vi "Arduino read multiple 10times resolution Feb2017.vi"(5 "# of points to average":i32, 8 "arduino addresses in":T2, 9 "average points?":bool, 10 "arduinos on?":bool) -> (1 "arduino addresses out":T2, 2 "freq out":T1, 3 "arduinos on":bool)   [LabVIEW 2014]
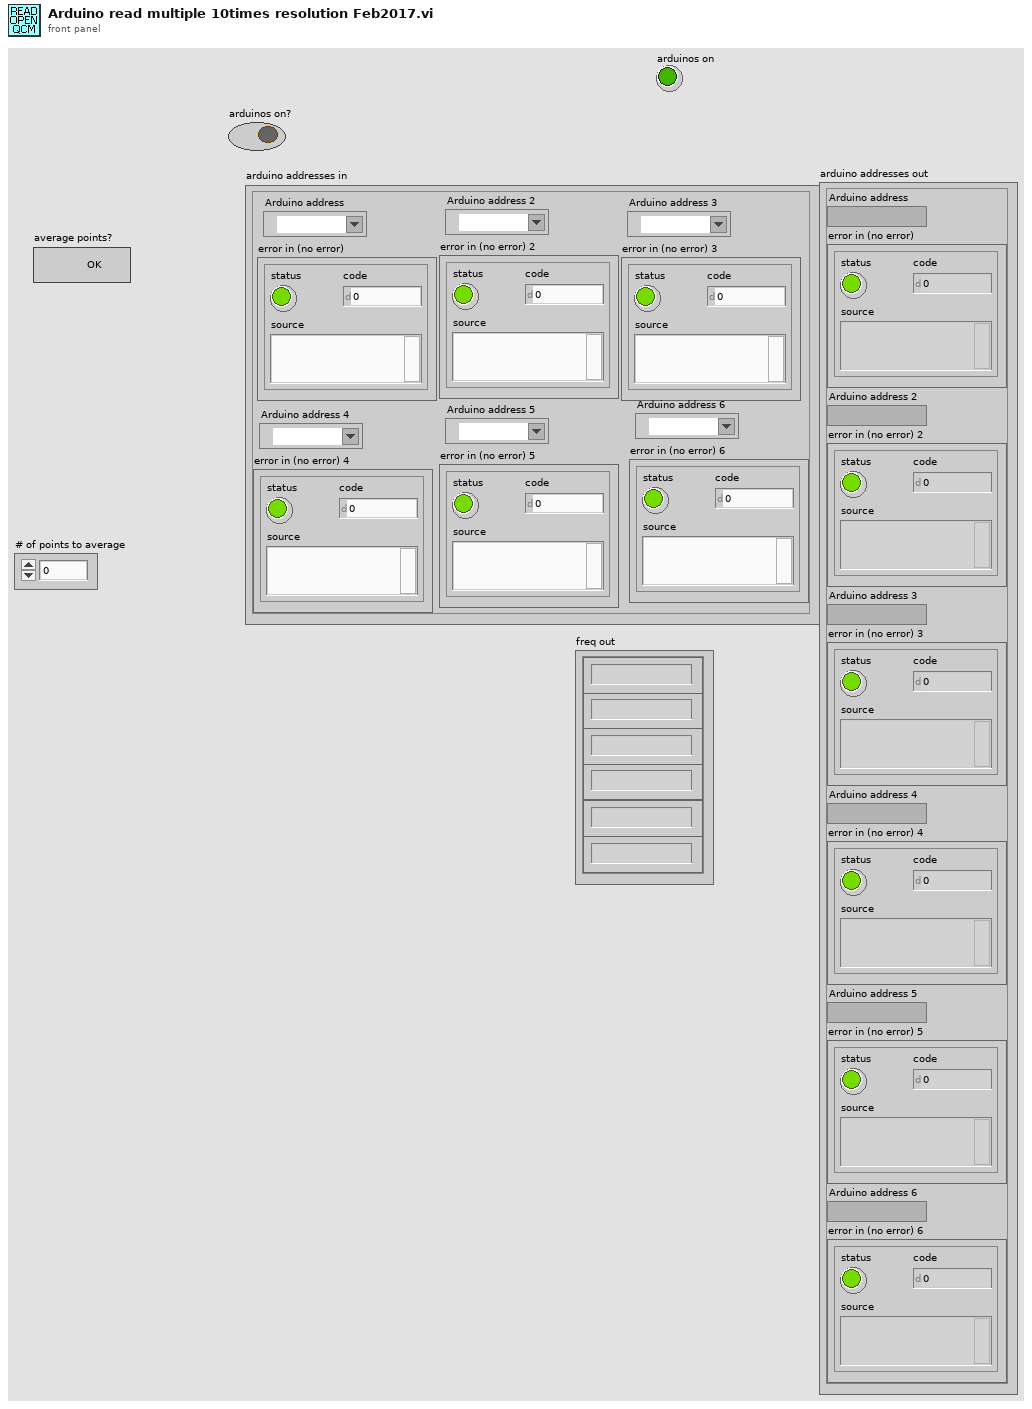
[diagram p1: front panel]
types:
  T1 = cluster{"String":string, "String":string, "String":string, "String":string, "String":string, "String":string}
  T2 = cluster{"Arduino address":refnum<visa-resource-name>, "error in (no error)":errorcluster, "Arduino address 2":refnum<visa-resource-name>, "error in (no error) 2":errorcluster, "Arduino address 3":refnum<visa-resource-name>, "error in (no error) 3":errorcluster, "Arduino address 4":refnum<visa-resource-name>, "error in (no error) 4":errorcluster, "Arduino address 5":refnum<visa-resource-name>, "error in (no error) 5":errorcluster, "Arduino address 6":refnum<visa-resource-name>, "error in (no error) 6":errorcluster}
  T3 = cluster{string, string, string, string, string, string}
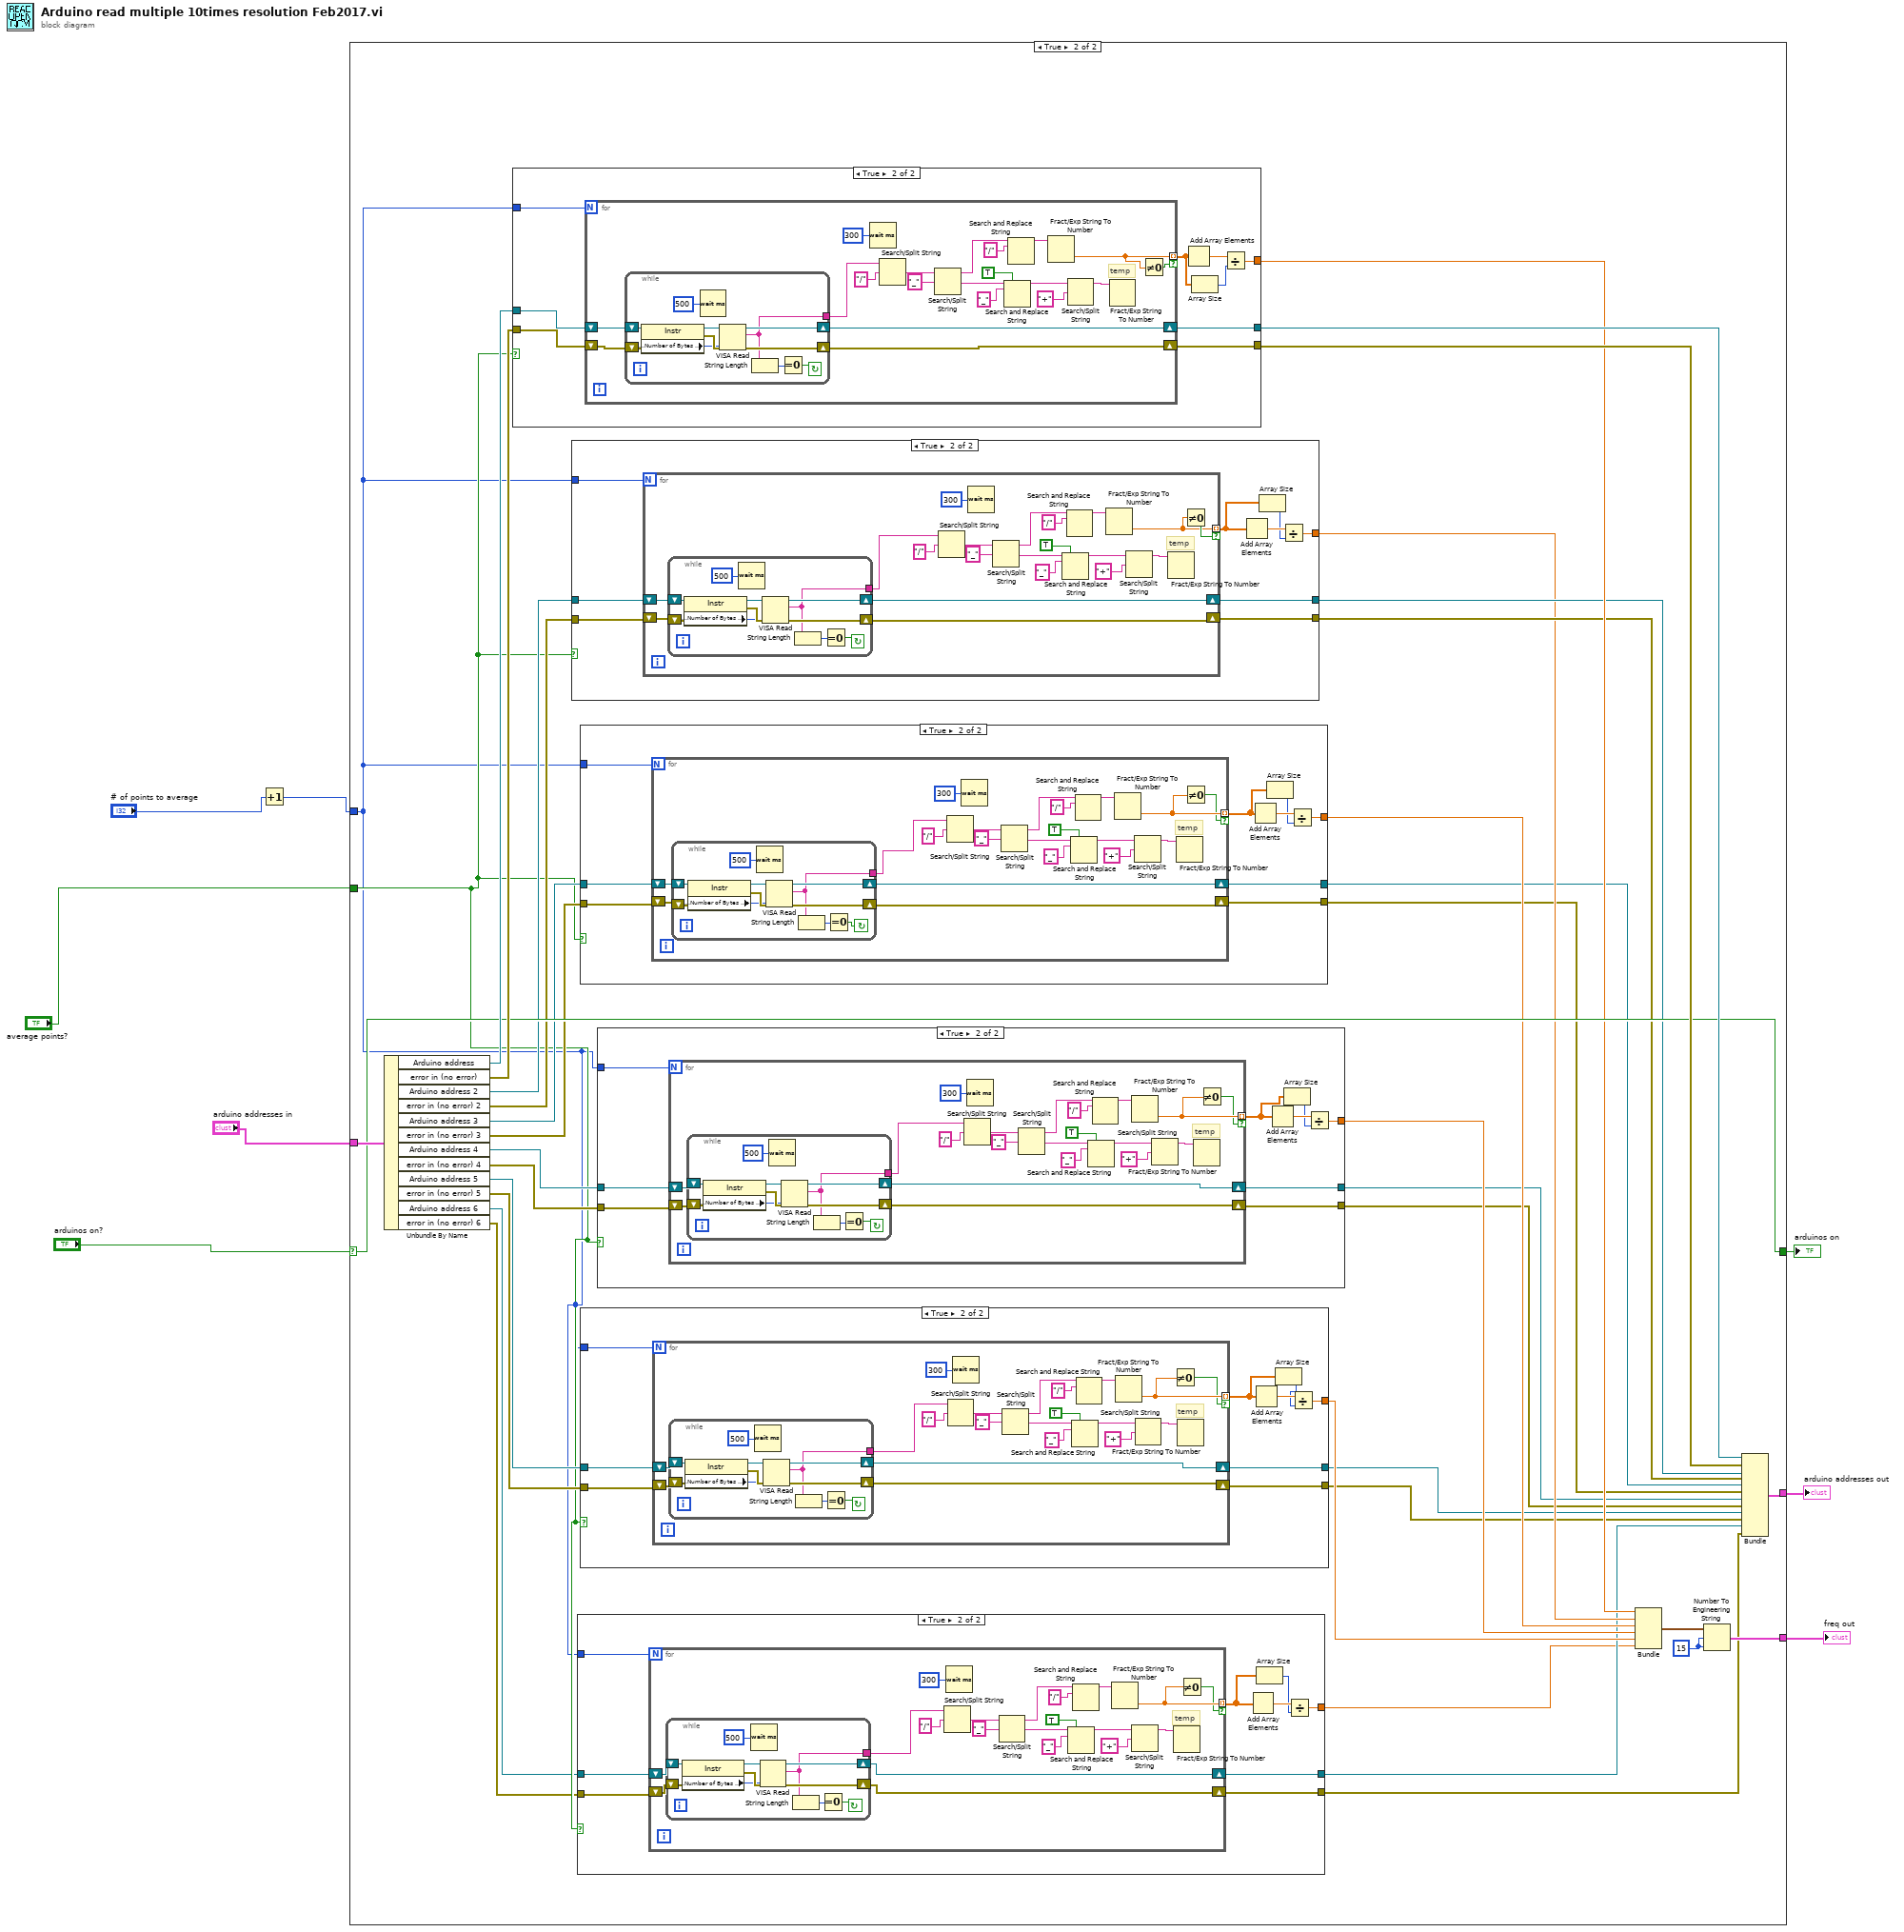
[diagram p0: block diagram]
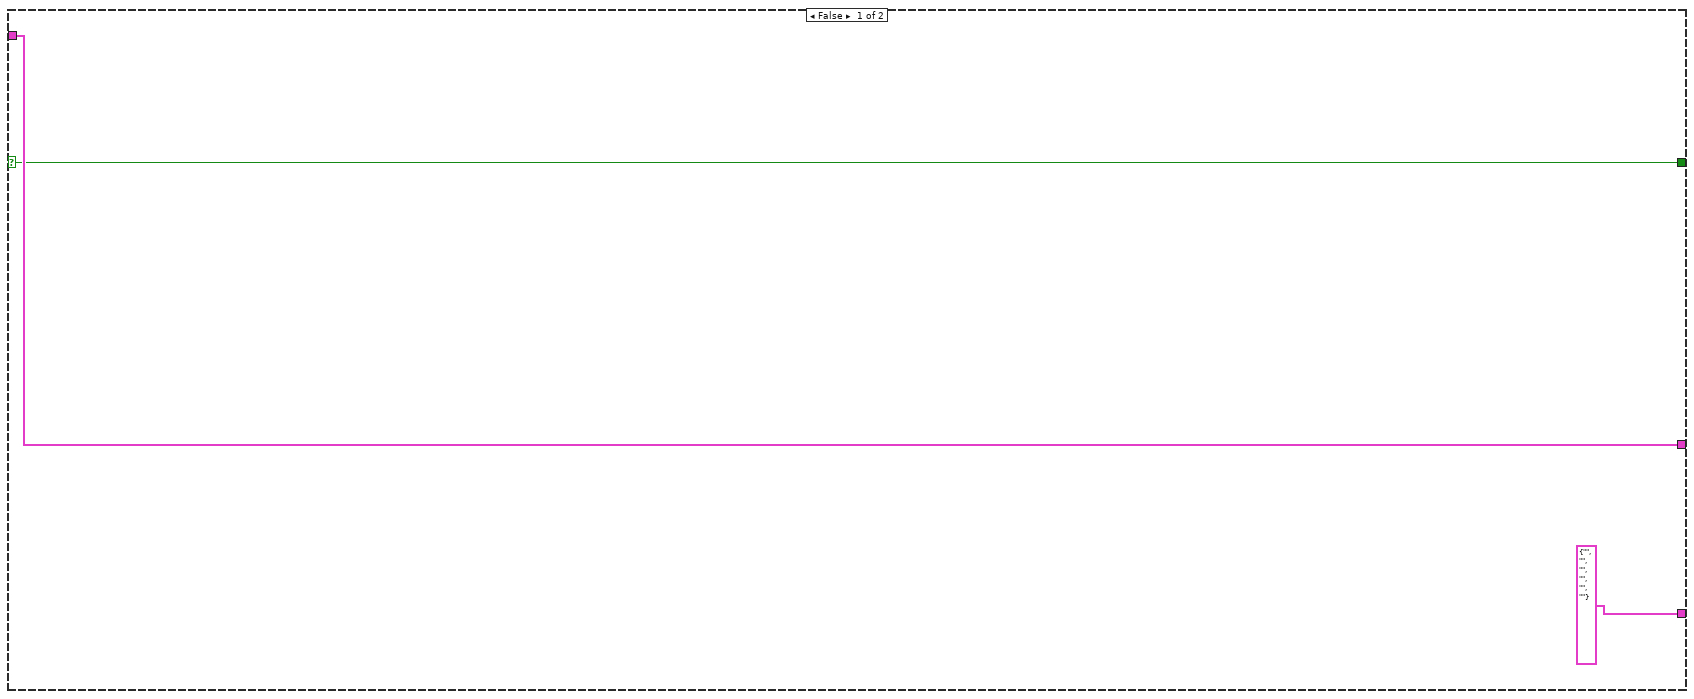
[diagram p2: hidden frame]
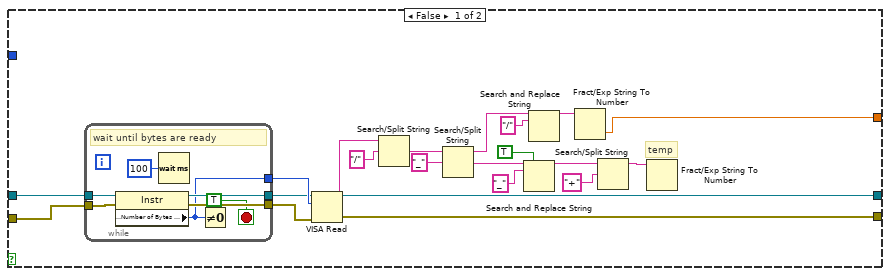
[diagram p3: hidden frame]
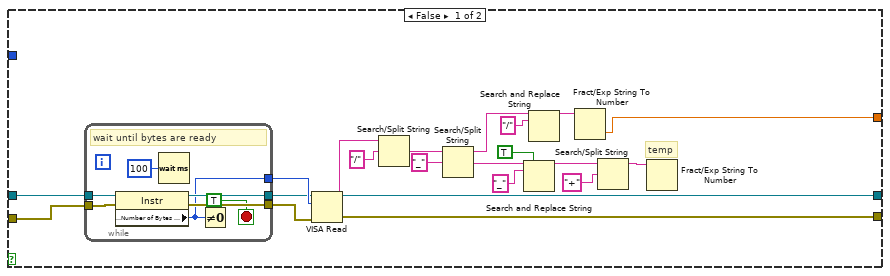
[diagram p4: hidden frame]
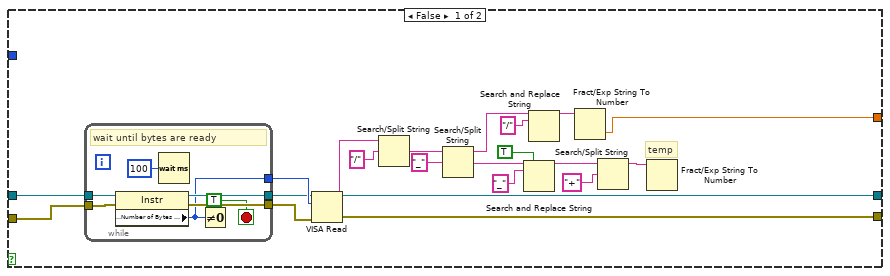
[diagram p5: hidden frame]
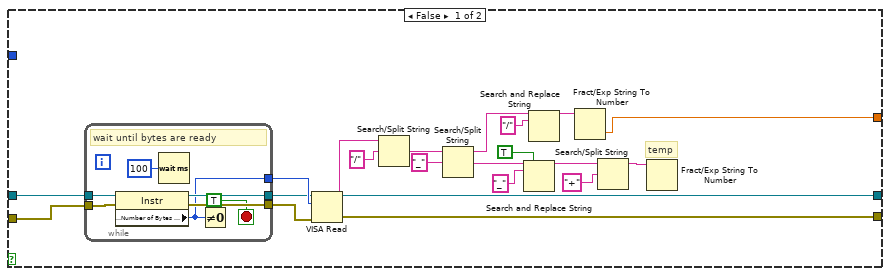
[diagram p6: hidden frame]
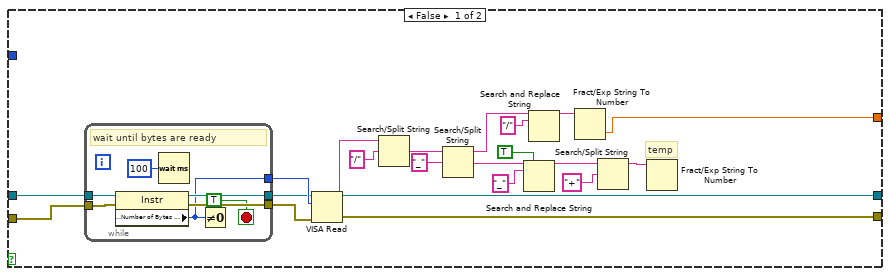
[diagram p7: hidden frame]
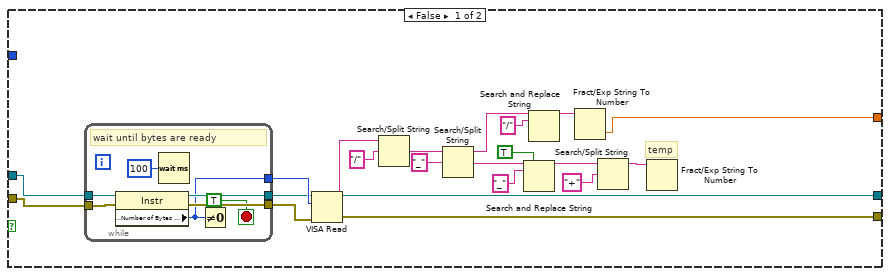
[diagram p8: hidden frame]
diagram:
  n1 = Increment(x="# of points to average") -> (x+1=w1:i32)
  n2 = case shown="True" "arduinos on?" {
    selector: "arduinos on?" -> [w10 w43]
    tunnel: "arduino addresses in" -> [w11 w49]
    tunnel: [w11 w44] -> w5
    tunnel: [w10 w43] -> w6
    tunnel: [T1 {"String"="", "String"="", "String"="", "String"="", "String"="", "String"=""} ("freq out") w40] -> w4
    tunnel: "average points?" -> [_ w18]
    tunnel: w1 -> [_ w17]
    frame False {
    }
    frame True {
      w42 = i16 15 ("width (-)")
      n3 = Unbundle By Name(w49) -> ("Arduino address"=w48:refnum<visa-resource-name>, "error in (no error)"=w47:errorcluster, "Arduino address 2"=w38:refnum<visa-resource-name>, "error in (no error) 2"=w37:errorcluster, "Arduino address 3"=w33:refnum<visa-resource-name>, "error in (no error) 3"=w32:errorcluster, "Arduino address 4"=w28:refnum<visa-resource-name>, "error in (no error) 4"=w27:errorcluster, "Arduino address 5"=w23:refnum<visa-resource-name>, "error in (no error) 5"=w22:errorcluster, "Arduino address 6"=w16:refnum<visa-resource-name>, "error in (no error) 6"=w15:errorcluster)
      n4 = case shown="True" w18 {
        tunnel: w48 -> [w394 w426]
        tunnel: w47 -> [w393 w425]
        tunnel: [w391 w424] -> w46
        tunnel: [w392 w423] -> w45
        tunnel: [w390 w421] -> w39
        tunnel: w17 -> [_ w418]
        frame False {
          # "temp"
          n5 = while {
            tunnel: w394 -> [w417]
            tunnel: [w416] -> w396
            tunnel: [w415] -> w395
            tunnel: [w414] -> w397
            tunnel: w393 -> [w411]
            stop <- TRUE stop-if-true
            # "wait until bytes are ready"
            n6 = property class="Instr"(reference=w417, error in=w411) -> (reference out=w415:refnum<visa-resource-name>, error out=w416:errorcluster, "Serial Settings:Number of Bytes at Serial Port"=w414:u32)
            n7 = Wait (ms)(milliseconds to wait=u32 100) -> ()  [unwired: 1 out]
            n8 = Not Equal To 0?(x=w414) -> ()  [unwired: 1 out]
          }
          n9 = VISA Read(VISA resource name=w395, byte count=w397, error in (no error)=w396) -> (VISA resource name out=w391:refnum<visa-resource-name>, read buffer=w410:string, error out=w392:errorcluster)  [unwired: 1 out]
          n10 = Search/Split String(string=w410, search string/char (-)="/") -> (match + rest of string=w403:string)  [unwired: 1 in, 2 out]
          n11 = Search/Split String(string=w403, search string/char (-)="_") -> (substring before match=w409:string, match + rest of string=w404:string)  [unwired: 1 in, 1 out]
          n12 = Search and Replace String(replace all?=TRUE ("replace all? (F)"), input string=w404, search string="_") -> (result string=w398:string)  [unwired: 5 in, 3 out]
          n13 = Search and Replace String(input string=w409, search string="/" ("replace string (\"\")")) -> (result string=w400:string)  [unwired: 6 in, 3 out]
          n14 = Fract/Exp String To Number(string=w400) -> (number=w390:dbl)  [unwired: 3 in, 1 out]
          n15 = Search/Split String(string=w398, search string/char (-)="+") -> (substring before match=w407:string)  [unwired: 1 in, 2 out]
          n16 = Fract/Exp String To Number(string=w407) -> ()  [unwired: 3 in, 2 out]
        }
        frame True {
          n17 = for {
            N: w418 -> [_]
            tunnel: [w432] -> w420 mode=indexing if=w431
            shift-right: [w434] -> w424
            shift-left: w426 -> [w430]
            shift-right: [w433] -> w423
            shift-left: w425 -> [w429]
            # "temp"
            n18 = while {
              shift-right: [w457] -> w434
              shift-left: w430 -> [w455]
              shift-right: [w456] -> w433
              shift-left: w429 -> [w454]
              tunnel: [w448] -> w427
              stop <- w449 continue-if-true
              n19 = property class="Instr"(reference=w455, error in=w454) -> (reference out=w452:refnum<visa-resource-name>, error out=w453:errorcluster, "Serial Settings:Number of Bytes at Serial Port"=w451:u32)
              n20 = Wait (ms)(milliseconds to wait=u32 500) -> ()  [unwired: 1 out]
              n21 = VISA Read(VISA resource name=w452, byte count=w451, error in (no error)=w453) -> (VISA resource name out=w457:refnum<visa-resource-name>, read buffer=w448:string, error out=w456:errorcluster)  [unwired: 1 out]
              n22 = String Length(string=w448) -> (length=w450:i32)
              n23 = Equal To 0?(x=w450) -> (x = 0?=w449:bool)
            }
            n24 = Wait (ms)(milliseconds to wait=u32 300) -> ()  [unwired: 1 out]
            n25 = Search/Split String(string=w427, search string/char (-)="/") -> (match + rest of string=w440:string)  [unwired: 1 in, 2 out]
            n26 = Search/Split String(string=w440, search string/char (-)="_") -> (substring before match=w446:string, match + rest of string=w441:string)  [unwired: 1 in, 1 out]
            n27 = Search and Replace String(replace all?=TRUE ("replace all? (F)"), input string=w441, search string="_") -> (result string=w435:string)  [unwired: 5 in, 3 out]
            n28 = Search and Replace String(input string=w446, search string="/" ("replace string (\"\")")) -> (result string=w437:string)  [unwired: 6 in, 3 out]
            n29 = Fract/Exp String To Number(string=w437) -> (number=w432:dbl)  [unwired: 3 in, 1 out]
            n30 = Search/Split String(string=w435, search string/char (-)="+") -> (substring before match=w444:string)  [unwired: 1 in, 2 out]
            n31 = Fract/Exp String To Number(string=w444) -> ()  [unwired: 3 in, 2 out]
            n32 = Not Equal To 0?(x=w432) -> (x != 0?=w431:bool)
          }
          n33 = Add Array Elements(numeric array=w420) -> (sum=w422:dbl)
          n34 = Array Size(array=w420) -> (size(s)=w419:i32)
          n35 = Divide(x=w422, y=w419) -> (x/y=w421:dbl)
        }
      }
      n36 = case shown="True" w18 {
        tunnel: w38 -> [w326 w358]
        tunnel: w37 -> [w325 w357]
        tunnel: [w323 w356] -> w36
        tunnel: [w324 w355] -> w35
        tunnel: [w322 w352] -> w34
        tunnel: w17 -> [_ w353]
        frame False {
          # "temp"
          n37 = while {
            tunnel: w326 -> [w349]
            tunnel: [w348] -> w328
            tunnel: [w347] -> w327
            tunnel: [w346] -> w329
            tunnel: w325 -> [w343]
            stop <- TRUE stop-if-true
            # "wait until bytes are ready"
            n38 = property class="Instr"(reference=w349, error in=w343) -> (reference out=w347:refnum<visa-resource-name>, error out=w348:errorcluster, "Serial Settings:Number of Bytes at Serial Port"=w346:u32)
            n39 = Wait (ms)(milliseconds to wait=u32 100) -> ()  [unwired: 1 out]
            n40 = Not Equal To 0?(x=w346) -> ()  [unwired: 1 out]
          }
          n41 = VISA Read(VISA resource name=w327, byte count=w329, error in (no error)=w328) -> (VISA resource name out=w323:refnum<visa-resource-name>, read buffer=w342:string, error out=w324:errorcluster)  [unwired: 1 out]
          n42 = Search/Split String(string=w342, search string/char (-)="/") -> (match + rest of string=w335:string)  [unwired: 1 in, 2 out]
          n43 = Search/Split String(string=w335, search string/char (-)="_") -> (substring before match=w341:string, match + rest of string=w336:string)  [unwired: 1 in, 1 out]
          n44 = Search and Replace String(replace all?=TRUE ("replace all? (F)"), input string=w336, search string="_") -> (result string=w330:string)  [unwired: 5 in, 3 out]
          n45 = Search and Replace String(input string=w341, search string="/" ("replace string (\"\")")) -> (result string=w332:string)  [unwired: 6 in, 3 out]
          n46 = Fract/Exp String To Number(string=w332) -> (number=w322:dbl)  [unwired: 3 in, 1 out]
          n47 = Search/Split String(string=w330, search string/char (-)="+") -> (substring before match=w339:string)  [unwired: 1 in, 2 out]
          n48 = Fract/Exp String To Number(string=w339) -> ()  [unwired: 3 in, 2 out]
        }
        frame True {
          n49 = for {
            N: w353 -> [_]
            tunnel: [w365] -> w350 mode=indexing if=w366
            shift-right: [w361] -> w356
            shift-left: w358 -> [w363]
            shift-right: [w360] -> w355
            shift-left: w357 -> [w362]
            # "temp"
            n50 = while {
              shift-right: [w389] -> w361
              shift-left: w363 -> [w387]
              shift-right: [w388] -> w360
              shift-left: w362 -> [w386]
              tunnel: [w380] -> w359
              stop <- w381 continue-if-true
              n51 = property class="Instr"(reference=w387, error in=w386) -> (reference out=w384:refnum<visa-resource-name>, error out=w385:errorcluster, "Serial Settings:Number of Bytes at Serial Port"=w383:u32)
              n52 = Wait (ms)(milliseconds to wait=u32 500) -> ()  [unwired: 1 out]
              n53 = VISA Read(VISA resource name=w384, byte count=w383, error in (no error)=w385) -> (VISA resource name out=w389:refnum<visa-resource-name>, read buffer=w380:string, error out=w388:errorcluster)  [unwired: 1 out]
              n54 = String Length(string=w380) -> (length=w382:i32)
              n55 = Equal To 0?(x=w382) -> (x = 0?=w381:bool)
            }
            n56 = Search/Split String(string=w359, search string/char (-)="/") -> (match + rest of string=w372:string)  [unwired: 1 in, 2 out]
            n57 = Wait (ms)(milliseconds to wait=u32 300) -> ()  [unwired: 1 out]
            n58 = Search/Split String(string=w372, search string/char (-)="_") -> (substring before match=w378:string, match + rest of string=w373:string)  [unwired: 1 in, 1 out]
            n59 = Search and Replace String(replace all?=TRUE ("replace all? (F)"), input string=w373, search string="_") -> (result string=w367:string)  [unwired: 5 in, 3 out]
            n60 = Search and Replace String(input string=w378, search string="/" ("replace string (\"\")")) -> (result string=w369:string)  [unwired: 6 in, 3 out]
            n61 = Fract/Exp String To Number(string=w369) -> (number=w365:dbl)  [unwired: 3 in, 1 out]
            n62 = Search/Split String(string=w367, search string/char (-)="+") -> (substring before match=w376:string)  [unwired: 1 in, 2 out]
            n63 = Fract/Exp String To Number(string=w376) -> ()  [unwired: 3 in, 2 out]
            n64 = Not Equal To 0?(x=w365) -> (x != 0?=w366:bool)
          }
          n65 = Add Array Elements(numeric array=w350) -> (sum=w354:dbl)
          n66 = Array Size(array=w350) -> (size(s)=w351:i32)
          n67 = Divide(x=w354, y=w351) -> (x/y=w352:dbl)
        }
      }
      n68 = case shown="True" w18 {
        tunnel: w16 -> [w54 w86]
        tunnel: w15 -> [w53 w85]
        tunnel: [w51 w84] -> w14
        tunnel: [w52 w83] -> w12
        tunnel: [w50 w80] -> w13
        tunnel: w17 -> [_ w81]
        frame False {
          # "temp"
          n69 = while {
            tunnel: w54 -> [w77]
            tunnel: [w76] -> w56
            tunnel: [w75] -> w55
            tunnel: [w74] -> w57
            tunnel: w53 -> [w71]
            stop <- TRUE stop-if-true
            # "wait until bytes are ready"
            n70 = property class="Instr"(reference=w77, error in=w71) -> (reference out=w75:refnum<visa-resource-name>, error out=w76:errorcluster, "Serial Settings:Number of Bytes at Serial Port"=w74:u32)
            n71 = Wait (ms)(milliseconds to wait=u32 100) -> ()  [unwired: 1 out]
            n72 = Not Equal To 0?(x=w74) -> ()  [unwired: 1 out]
          }
          n73 = VISA Read(VISA resource name=w55, byte count=w57, error in (no error)=w56) -> (VISA resource name out=w51:refnum<visa-resource-name>, read buffer=w70:string, error out=w52:errorcluster)  [unwired: 1 out]
          n74 = Search/Split String(string=w70, search string/char (-)="/") -> (match + rest of string=w63:string)  [unwired: 1 in, 2 out]
          n75 = Search/Split String(string=w63, search string/char (-)="_") -> (substring before match=w69:string, match + rest of string=w64:string)  [unwired: 1 in, 1 out]
          n76 = Search and Replace String(replace all?=TRUE ("replace all? (F)"), input string=w64, search string="_") -> (result string=w58:string)  [unwired: 5 in, 3 out]
          n77 = Search and Replace String(input string=w69, search string="/" ("replace string (\"\")")) -> (result string=w60:string)  [unwired: 6 in, 3 out]
          n78 = Fract/Exp String To Number(string=w60) -> (number=w50:dbl)  [unwired: 3 in, 1 out]
          n79 = Search/Split String(string=w58, search string/char (-)="+") -> (substring before match=w67:string)  [unwired: 1 in, 2 out]
          n80 = Fract/Exp String To Number(string=w67) -> ()  [unwired: 3 in, 2 out]
        }
        frame True {
          n81 = for {
            N: w81 -> [_]
            tunnel: [w94] -> w78 mode=indexing if=w93
            shift-right: [w88] -> w84
            shift-left: w86 -> [w91]
            shift-right: [w87] -> w83
            shift-left: w85 -> [w90]
            # "temp"
            n82 = while {
              shift-right: [w117] -> w88
              shift-left: w91 -> [w115]
              shift-right: [w116] -> w87
              shift-left: w90 -> [w114]
              tunnel: [w108] -> w89
              stop <- w109 continue-if-true
              n83 = property class="Instr"(reference=w115, error in=w114) -> (reference out=w112:refnum<visa-resource-name>, error out=w113:errorcluster, "Serial Settings:Number of Bytes at Serial Port"=w111:u32)
              n84 = Wait (ms)(milliseconds to wait=u32 500) -> ()  [unwired: 1 out]
              n85 = VISA Read(VISA resource name=w112, byte count=w111, error in (no error)=w113) -> (VISA resource name out=w117:refnum<visa-resource-name>, read buffer=w108:string, error out=w116:errorcluster)  [unwired: 1 out]
              n86 = String Length(string=w108) -> (length=w110:i32)
              n87 = Equal To 0?(x=w110) -> (x = 0?=w109:bool)
            }
            n88 = Search/Split String(string=w89, search string/char (-)="/") -> (match + rest of string=w100:string)  [unwired: 1 in, 2 out]
            n89 = Wait (ms)(milliseconds to wait=u32 300) -> ()  [unwired: 1 out]
            n90 = Search/Split String(string=w100, search string/char (-)="_") -> (substring before match=w106:string, match + rest of string=w101:string)  [unwired: 1 in, 1 out]
            n91 = Search and Replace String(replace all?=TRUE ("replace all? (F)"), input string=w101, search string="_") -> (result string=w95:string)  [unwired: 5 in, 3 out]
            n92 = Search and Replace String(input string=w106, search string="/" ("replace string (\"\")")) -> (result string=w97:string)  [unwired: 6 in, 3 out]
            n93 = Fract/Exp String To Number(string=w97) -> (number=w94:dbl)  [unwired: 3 in, 1 out]
            n94 = Search/Split String(string=w95, search string/char (-)="+") -> (substring before match=w104:string)  [unwired: 1 in, 2 out]
            n95 = Fract/Exp String To Number(string=w104) -> ()  [unwired: 3 in, 2 out]
            n96 = Not Equal To 0?(x=w94) -> (x != 0?=w93:bool)
          }
          n97 = Add Array Elements(numeric array=w78) -> (sum=w82:dbl)
          n98 = Array Size(array=w78) -> (size(s)=w79:i32)
          n99 = Divide(x=w82, y=w79) -> (x/y=w80:dbl)
        }
      }
      n100 = case shown="True" w18 {
        tunnel: w33 -> [w258 w290]
        tunnel: w32 -> [w257 w289]
        tunnel: [w255 w288] -> w29
        tunnel: [w256 w287] -> w30
        tunnel: [w254 w285] -> w31
        tunnel: w17 -> [_ w283]
        frame False {
          # "temp"
          n101 = while {
            tunnel: w258 -> [w281]
            tunnel: [w280] -> w260
            tunnel: [w279] -> w259
            tunnel: [w278] -> w261
            tunnel: w257 -> [w275]
            stop <- TRUE stop-if-true
            # "wait until bytes are ready"
            n102 = property class="Instr"(reference=w281, error in=w275) -> (reference out=w279:refnum<visa-resource-name>, error out=w280:errorcluster, "Serial Settings:Number of Bytes at Serial Port"=w278:u32)
            n103 = Wait (ms)(milliseconds to wait=u32 100) -> ()  [unwired: 1 out]
            n104 = Not Equal To 0?(x=w278) -> ()  [unwired: 1 out]
          }
          n105 = VISA Read(VISA resource name=w259, byte count=w261, error in (no error)=w260) -> (VISA resource name out=w255:refnum<visa-resource-name>, read buffer=w274:string, error out=w256:errorcluster)  [unwired: 1 out]
          n106 = Search/Split String(string=w274, search string/char (-)="/") -> (match + rest of string=w267:string)  [unwired: 1 in, 2 out]
          n107 = Search/Split String(string=w267, search string/char (-)="_") -> (substring before match=w273:string, match + rest of string=w268:string)  [unwired: 1 in, 1 out]
          n108 = Search and Replace String(replace all?=TRUE ("replace all? (F)"), input string=w268, search string="_") -> (result string=w262:string)  [unwired: 5 in, 3 out]
          n109 = Search and Replace String(input string=w273, search string="/" ("replace string (\"\")")) -> (result string=w264:string)  [unwired: 6 in, 3 out]
          n110 = Fract/Exp String To Number(string=w264) -> (number=w254:dbl)  [unwired: 3 in, 1 out]
          n111 = Search/Split String(string=w262, search string/char (-)="+") -> (substring before match=w271:string)  [unwired: 1 in, 2 out]
          n112 = Fract/Exp String To Number(string=w271) -> ()  [unwired: 3 in, 2 out]
        }
        frame True {
          n113 = for {
            N: w283 -> [_]
            tunnel: [w298] -> w284 mode=indexing if=w297
            shift-right: [w292] -> w288
            shift-left: w290 -> [w295]
            shift-right: [w291] -> w287
            shift-left: w289 -> [w294]
            # "temp"
            n114 = while {
              shift-right: [w321] -> w292
              shift-left: w295 -> [w319]
              shift-right: [w320] -> w291
              shift-left: w294 -> [w318]
              tunnel: [w312] -> w293
              stop <- w313 continue-if-true
              n115 = property class="Instr"(reference=w319, error in=w318) -> (reference out=w316:refnum<visa-resource-name>, error out=w317:errorcluster, "Serial Settings:Number of Bytes at Serial Port"=w315:u32)
              n116 = Wait (ms)(milliseconds to wait=u32 500) -> ()  [unwired: 1 out]
              n117 = VISA Read(VISA resource name=w316, byte count=w315, error in (no error)=w317) -> (VISA resource name out=w321:refnum<visa-resource-name>, read buffer=w312:string, error out=w320:errorcluster)  [unwired: 1 out]
              n118 = String Length(string=w312) -> (length=w314:i32)
              n119 = Equal To 0?(x=w314) -> (x = 0?=w313:bool)
            }
            n120 = Search/Split String(string=w293, search string/char (-)="/") -> (match + rest of string=w304:string)  [unwired: 1 in, 2 out]
            n121 = Wait (ms)(milliseconds to wait=u32 300) -> ()  [unwired: 1 out]
            n122 = Search/Split String(string=w304, search string/char (-)="_") -> (substring before match=w310:string, match + rest of string=w305:string)  [unwired: 1 in, 1 out]
            n123 = Search and Replace String(replace all?=TRUE ("replace all? (F)"), input string=w305, search string="_") -> (result string=w299:string)  [unwired: 5 in, 3 out]
            n124 = Search and Replace String(input string=w310, search string="/" ("replace string (\"\")")) -> (result string=w301:string)  [unwired: 6 in, 3 out]
            n125 = Fract/Exp String To Number(string=w301) -> (number=w298:dbl)  [unwired: 3 in, 1 out]
            n126 = Search/Split String(string=w299, search string/char (-)="+") -> (substring before match=w308:string)  [unwired: 1 in, 2 out]
            n127 = Fract/Exp String To Number(string=w308) -> ()  [unwired: 3 in, 2 out]
            n128 = Not Equal To 0?(x=w298) -> (x != 0?=w297:bool)
          }
          n129 = Add Array Elements(numeric array=w284) -> (sum=w286:dbl)
          n130 = Array Size(array=w284) -> (size(s)=w282:i32)
          n131 = Divide(x=w286, y=w282) -> (x/y=w285:dbl)
        }
      }
      n132 = case shown="True" w18 {
        tunnel: w23 -> [w122 w154]
        tunnel: w22 -> [w121 w153]
        tunnel: [w119 w152] -> w20
        tunnel: [w120 w151] -> w19
        tunnel: [w118 w148] -> w21
        tunnel: w17 -> [_ w149]
        frame False {
          # "temp"
          n133 = while {
            tunnel: w122 -> [w145]
            tunnel: [w144] -> w124
            tunnel: [w143] -> w123
            tunnel: [w142] -> w125
            tunnel: w121 -> [w139]
            stop <- TRUE stop-if-true
            # "wait until bytes are ready"
            n134 = property class="Instr"(reference=w145, error in=w139) -> (reference out=w143:refnum<visa-resource-name>, error out=w144:errorcluster, "Serial Settings:Number of Bytes at Serial Port"=w142:u32)
            n135 = Wait (ms)(milliseconds to wait=u32 100) -> ()  [unwired: 1 out]
            n136 = Not Equal To 0?(x=w142) -> ()  [unwired: 1 out]
          }
          n137 = VISA Read(VISA resource name=w123, byte count=w125, error in (no error)=w124) -> (VISA resource name out=w119:refnum<visa-resource-name>, read buffer=w138:string, error out=w120:errorcluster)  [unwired: 1 out]
          n138 = Search/Split String(string=w138, search string/char (-)="/") -> (match + rest of string=w131:string)  [unwired: 1 in, 2 out]
          n139 = Search/Split String(string=w131, search string/char (-)="_") -> (substring before match=w137:string, match + rest of string=w132:string)  [unwired: 1 in, 1 out]
          n140 = Search and Replace String(replace all?=TRUE ("replace all? (F)"), input string=w132, search string="_") -> (result string=w126:string)  [unwired: 5 in, 3 out]
          n141 = Search and Replace String(input string=w137, search string="/" ("replace string (\"\")")) -> (result string=w128:string)  [unwired: 6 in, 3 out]
          n142 = Fract/Exp String To Number(string=w128) -> (number=w118:dbl)  [unwired: 3 in, 1 out]
          n143 = Search/Split String(string=w126, search string/char (-)="+") -> (substring before match=w135:string)  [unwired: 1 in, 2 out]
          n144 = Fract/Exp String To Number(string=w135) -> ()  [unwired: 3 in, 2 out]
        }
        frame True {
          n145 = for {
            N: w149 -> [_]
            tunnel: [w162] -> w146 mode=indexing if=w161
            shift-right: [w157] -> w152
            shift-left: w154 -> [w159]
            shift-right: [w156] -> w151
            shift-left: w153 -> [w158]
            # "temp"
            n146 = while {
              shift-right: [w185] -> w157
              shift-left: w159 -> [w183]
              shift-right: [w184] -> w156
              shift-left: w158 -> [w182]
              tunnel: [w176] -> w155
              stop <- w177 continue-if-true
              n147 = property class="Instr"(reference=w183, error in=w182) -> (reference out=w180:refnum<visa-resource-name>, error out=w181:errorcluster, "Serial Settings:Number of Bytes at Serial Port"=w179:u32)
              n148 = Wait (ms)(milliseconds to wait=u32 500) -> ()  [unwired: 1 out]
              n149 = VISA Read(VISA resource name=w180, byte count=w179, error in (no error)=w181) -> (VISA resource name out=w185:refnum<visa-resource-name>, read buffer=w176:string, error out=w184:errorcluster)  [unwired: 1 out]
              n150 = String Length(string=w176) -> (length=w178:i32)
              n151 = Equal To 0?(x=w178) -> (x = 0?=w177:bool)
            }
            n152 = Search/Split String(string=w155, search string/char (-)="/") -> (match + rest of string=w168:string)  [unwired: 1 in, 2 out]
            n153 = Wait (ms)(milliseconds to wait=u32 300) -> ()  [unwired: 1 out]
            n154 = Search/Split String(string=w168, search string/char (-)="_") -> (substring before match=w174:string, match + rest of string=w169:string)  [unwired: 1 in, 1 out]
            n155 = Search and Replace String(replace all?=TRUE ("replace all? (F)"), input string=w169, search string="_") -> (result string=w163:string)  [unwired: 5 in, 3 out]
            n156 = Search and Replace String(input string=w174, search string="/" ("replace string (\"\")")) -> (result string=w165:string)  [unwired: 6 in, 3 out]
            n157 = Fract/Exp String To Number(string=w165) -> (number=w162:dbl)  [unwired: 3 in, 1 out]
            n158 = Search/Split String(string=w163, search string/char (-)="+") -> (substring before match=w172:string)  [unwired: 1 in, 2 out]
            n159 = Not Equal To 0?(x=w162) -> (x != 0?=w161:bool)
            n160 = Fract/Exp String To Number(string=w172) -> ()  [unwired: 3 in, 2 out]
          }
          n161 = Add Array Elements(numeric array=w146) -> (sum=w150:dbl)
          n162 = Array Size(array=w146) -> (size(s)=w147:i32)
          n163 = Divide(x=w150, y=w147) -> (x/y=w148:dbl)
        }
      }
      n164 = case shown="True" w18 {
        tunnel: w28 -> [w190 w222]
        tunnel: w27 -> [w189 w221]
        tunnel: [w187 w220] -> w25
        tunnel: [w188 w219] -> w24
        tunnel: [w186 w216] -> w26
        tunnel: w17 -> [_ w217]
        frame False {
          # "temp"
          n165 = while {
            tunnel: w190 -> [w213]
            tunnel: [w212] -> w192
            tunnel: [w211] -> w191
            tunnel: [w210] -> w193
            tunnel: w189 -> [w207]
            stop <- TRUE stop-if-true
            # "wait until bytes are ready"
            n166 = property class="Instr"(reference=w213, error in=w207) -> (reference out=w211:refnum<visa-resource-name>, error out=w212:errorcluster, "Serial Settings:Number of Bytes at Serial Port"=w210:u32)
            n167 = Wait (ms)(milliseconds to wait=u32 100) -> ()  [unwired: 1 out]
            n168 = Not Equal To 0?(x=w210) -> ()  [unwired: 1 out]
          }
          n169 = VISA Read(VISA resource name=w191, byte count=w193, error in (no error)=w192) -> (VISA resource name out=w187:refnum<visa-resource-name>, read buffer=w206:string, error out=w188:errorcluster)  [unwired: 1 out]
          n170 = Search/Split String(string=w206, search string/char (-)="/") -> (match + rest of string=w199:string)  [unwired: 1 in, 2 out]
          n171 = Search/Split String(string=w199, search string/char (-)="_") -> (substring before match=w205:string, match + rest of string=w200:string)  [unwired: 1 in, 1 out]
          n172 = Search and Replace String(replace all?=TRUE ("replace all? (F)"), input string=w200, search string="_") -> (result string=w194:string)  [unwired: 5 in, 3 out]
          n173 = Search and Replace String(input string=w205, search string="/" ("replace string (\"\")")) -> (result string=w196:string)  [unwired: 6 in, 3 out]
          n174 = Fract/Exp String To Number(string=w196) -> (number=w186:dbl)  [unwired: 3 in, 1 out]
          n175 = Search/Split String(string=w194, search string/char (-)="+") -> (substring before match=w203:string)  [unwired: 1 in, 2 out]
          n176 = Fract/Exp String To Number(string=w203) -> ()  [unwired: 3 in, 2 out]
        }
        frame True {
          n177 = for {
            N: w217 -> [_]
            tunnel: [w230] -> w214 mode=indexing if=w229
            shift-right: [w225] -> w220
            shift-left: w222 -> [w227]
            shift-right: [w224] -> w219
            shift-left: w221 -> [w226]
            # "temp"
            n178 = while {
              shift-right: [w253] -> w225
              shift-left: w227 -> [w251]
              shift-right: [w252] -> w224
              shift-left: w226 -> [w250]
              tunnel: [w244] -> w223
              stop <- w245 continue-if-true
              n179 = property class="Instr"(reference=w251, error in=w250) -> (reference out=w248:refnum<visa-resource-name>, error out=w249:errorcluster, "Serial Settings:Number of Bytes at Serial Port"=w247:u32)
              n180 = Wait (ms)(milliseconds to wait=u32 500) -> ()  [unwired: 1 out]
              n181 = VISA Read(VISA resource name=w248, byte count=w247, error in (no error)=w249) -> (VISA resource name out=w253:refnum<visa-resource-name>, read buffer=w244:string, error out=w252:errorcluster)  [unwired: 1 out]
              n182 = String Length(string=w244) -> (length=w246:i32)
              n183 = Equal To 0?(x=w246) -> (x = 0?=w245:bool)
            }
            n184 = Search/Split String(string=w223, search string/char (-)="/") -> (match + rest of string=w236:string)  [unwired: 1 in, 2 out]
            n185 = Wait (ms)(milliseconds to wait=u32 300) -> ()  [unwired: 1 out]
            n186 = Search/Split String(string=w236, search string/char (-)="_") -> (substring before match=w242:string, match + rest of string=w237:string)  [unwired: 1 in, 1 out]
            n187 = Search and Replace String(replace all?=TRUE ("replace all? (F)"), input string=w237, search string="_") -> (result string=w231:string)  [unwired: 5 in, 3 out]
            n188 = Search and Replace String(input string=w242, search string="/" ("replace string (\"\")")) -> (result string=w233:string)  [unwired: 6 in, 3 out]
            n189 = Fract/Exp String To Number(string=w233) -> (number=w230:dbl)  [unwired: 3 in, 1 out]
            n190 = Search/Split String(string=w231, search string/char (-)="+") -> (substring before match=w240:string)  [unwired: 1 in, 2 out]
            n191 = Fract/Exp String To Number(string=w240) -> ()  [unwired: 3 in, 2 out]
            n192 = Not Equal To 0?(x=w230) -> (x != 0?=w229:bool)
          }
          n193 = Add Array Elements(numeric array=w214) -> (sum=w218:dbl)
          n194 = Array Size(array=w214) -> (size(s)=w215:i32)
          n195 = Divide(x=w218, y=w215) -> (x/y=w216:dbl)
        }
      }
      n196 = Bundle(w39, w34, w31, w26, w21, w13) -> (w41:cluster{dbl, dbl, dbl, dbl, dbl, dbl})  [unwired: 1 in]
      n197 = Number To Engineering String(2:w42, 3:w42, 4:w41) -> (0:w40:T3)  [unwired: 1 in]
      n198 = Bundle("Arduino address"=w46, "error in (no error)"=w45, "Arduino address 2"=w36, "error in (no error) 2"=w35, "Arduino address 3"=w29, "error in (no error) 3"=w30, "Arduino address 4"=w25, "error in (no error) 4"=w24, "Arduino address 5"=w20, "error in (no error) 5"=w19, "Arduino address 6"=w14, "error in (no error) 6"=w12) -> (w44:T2)  [unwired: 1 in]
    }
  }
  "arduinos on" <- w6
  "arduino addresses out" <- w5
  "freq out" <- w4
